vi "2021 Advent puzzle 05 Add via lines new.vi"(6 "Y2":i32[](array[numeric]), 8 "X2":i32[](array[numeric]), 9 "Y1":i32[](array[numeric]), 10 "X1":i32[](array[numeric]), 11 "Array in":i16[][](array[numeric])) -> (3 "Array out":i16[][](array[numeric]))   [LabVIEW 2021]
panel:
  in  "index":i32
  out "Array out 4":i16[][](array[numeric])
  out "Loop":i32
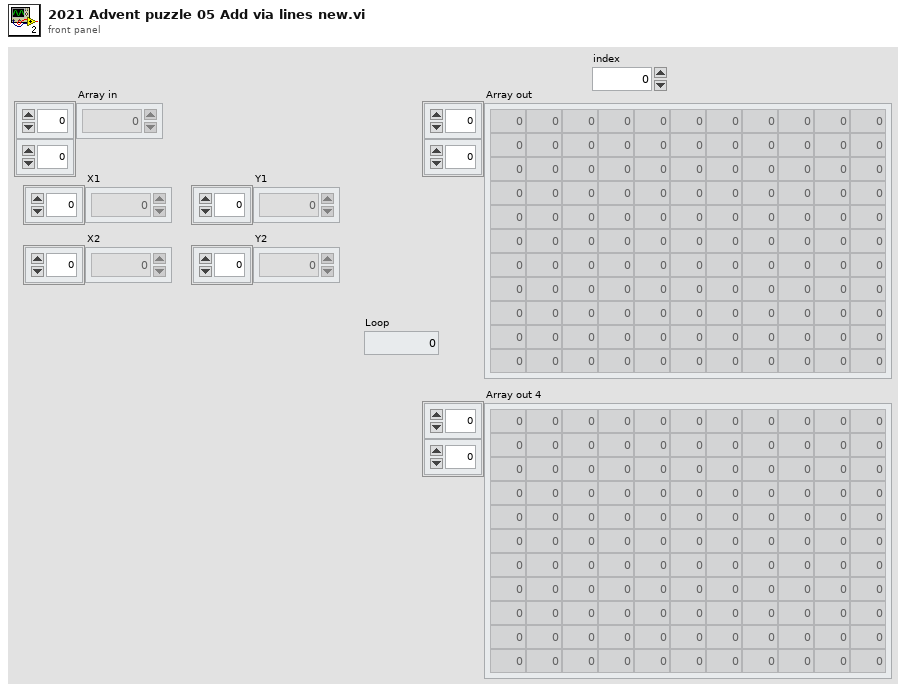
[diagram p1: front panel]
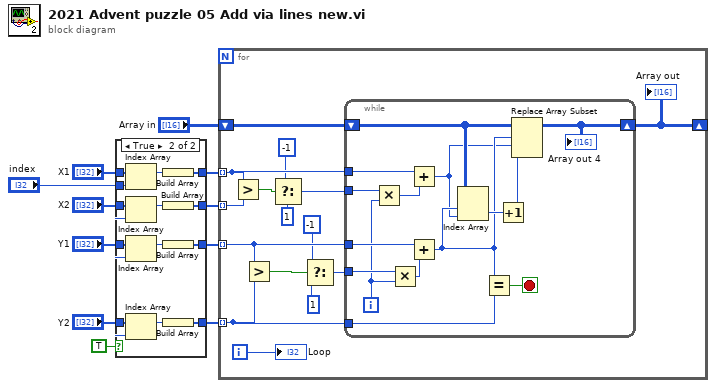
[diagram p0: block diagram]
diagram:
  n1 = case shown="True" TRUE {
    tunnel: "Y2" -> [w12 w28]
    tunnel: "Y1" -> [w13 w27]
    tunnel: "X2" -> [w14 w26]
    tunnel: "X1" -> [w15 w25]
    tunnel: [w15 w23] -> w6
    tunnel: [w14 w19] -> w5
    tunnel: [w13 w18] -> w4
    tunnel: [w12 w17] -> w3
    tunnel: "index" -> [_ w16]
    frame False {
    }
    frame True {
      n2 = Index Array(array=w25, index=w16) -> (element=w24:i32)
      n3 = Index Array(array=w26, index=w16) -> (element=w22:i32)
      n4 = Index Array(array=w27, index=w16) -> (element=w21:i32)
      n5 = Index Array(array=w28, index=w16) -> (element=w20:i32)
      n6 = Build Array(w24) -> (w23:i32[])
      n7 = Build Array(w22) -> (w19:i32[])
      n8 = Build Array(w21) -> (w18:i32[])
      n9 = Build Array(w20) -> (w17:i32[])
    }
  }
  n10 = for {
    tunnel: w6 -> [w41] mode=indexing
    tunnel: w5 -> [w43] mode=indexing
    tunnel: w4 -> [w42] mode=indexing
    tunnel: w3 -> [w40] mode=indexing
    shift-right: [w38] -> _
    shift-left: "Array in" -> [w39]
    i -> [w37]
    n11 = Greater?(x=w41, y=w43) -> (0:w36:bool)
    n12 = Greater?(x=w42, y=w40) -> (0:w29:bool)
    n13 = Select(t=-1, s=w36, f=1) -> (s? t:f=w33:i32)
    n14 = Select(t=-1, s=w29, f=1) -> (s? t:f=w30:i32)
    n15 = while {
      shift-right: [w57] -> w38
      shift-left: w39 -> [w58]
      tunnel: w41 -> [w54]
      tunnel: w42 -> [w55]
      tunnel: w40 -> [w52]
      tunnel: w33 -> [w50]
      tunnel: w30 -> [w49]
      i -> [w46]
      stop <- w51 stop-if-true
      n16 = Multiply(x=w50, y=w46) -> (x*y=w47:i32)
      n17 = Multiply(x=w49, y=w46) -> (x*y=w48:i32)
      n18 = Add(x=w54, y=w47) -> (x+y=w44:i32)
      n19 = Add(x=w55, y=w48) -> (x+y=w45:i32)
      n20 = Index Array(array=w58, index (row)=w45, index (col)=w44) -> (element=w56:i16)
      n21 = Equal?(x=w45, y=w52) -> (x = y?=w51:bool)
      n22 = Increment(x=w56) -> (x+1=w53:i16)
      n23 = Replace Array Subset(array=w58, new element=w53, index (row)=w45, index (col)=w44) -> (w57:i16[][])
      "Array out 4" <- w57
    }
    "Array out" <- w38
    "Loop" <- w37
  }
